vi "Run.vi"(8 "error in (no error)":errorcluster, 11 "Car Wash Station Sequencer in":refnum<class "Car Wash Station Sequencer.lvclass">) -> (0 "error out":errorcluster, 3 "Car Wash Station Sequencer out":refnum<class "Car Wash Station Sequencer.lvclass">)   [LabVIEW 2016, in "CLD Exam - Car Wash.lvlib" / "Car Wash Station Sequencer.lvclass"]
doc: "--\nCopyright © 2017 Composed SystemsI All rights reserved.\n\nAuthor: Jon McBee <jon.mcbee@composed.io>\n\nThis library is provided \"AS IS\" ,WITHOUT WARRANTIES OR\nCONDITIONS OF ANY KIND, either express or implied.\n\nComposed Systems -- composed.io\n\nStream 0.0.1.1\nJon McBee - Composed Systems\nCopyright (c) 2017, Composed Systems"
uses:
  Car Wash Station Sequencer.lvclass
  D:/Repos/Stream/software/Mediator/Classes/Mediated Actor/Mediated Actor.lvclass
  Mediator/Classes/Message Interface/Message Interface.lvclass
  Car Wash Station Sequencer.lvclass/Car Wash Station Sequencer.ctl
  Car Wash Started Event/Car Wash Started.lvclass
  Car Position Changed Event/Car Position Changed.lvclass
  Mediator/Classes/Mediated Actor/Mediated Actor.lvclass
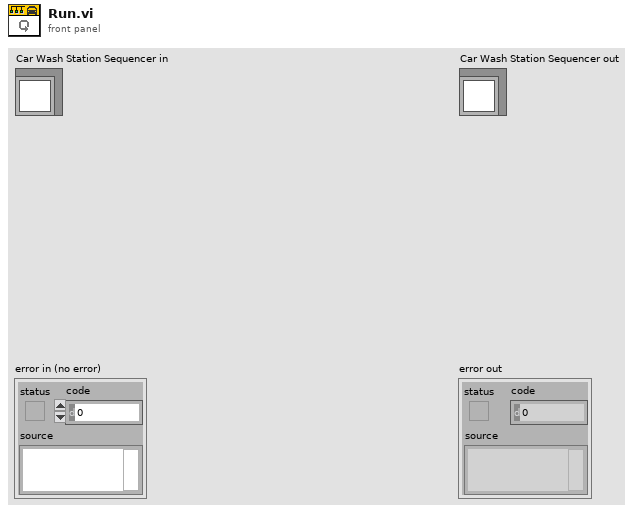
[diagram p1: front panel]
types:
  T1 = cluster{"System Exit":refnum<event-registration>, "To Self":refnum<event-registration>, "Car Wash Started":refnum<event-registration>, "Car Position Changed":refnum<event-registration>}
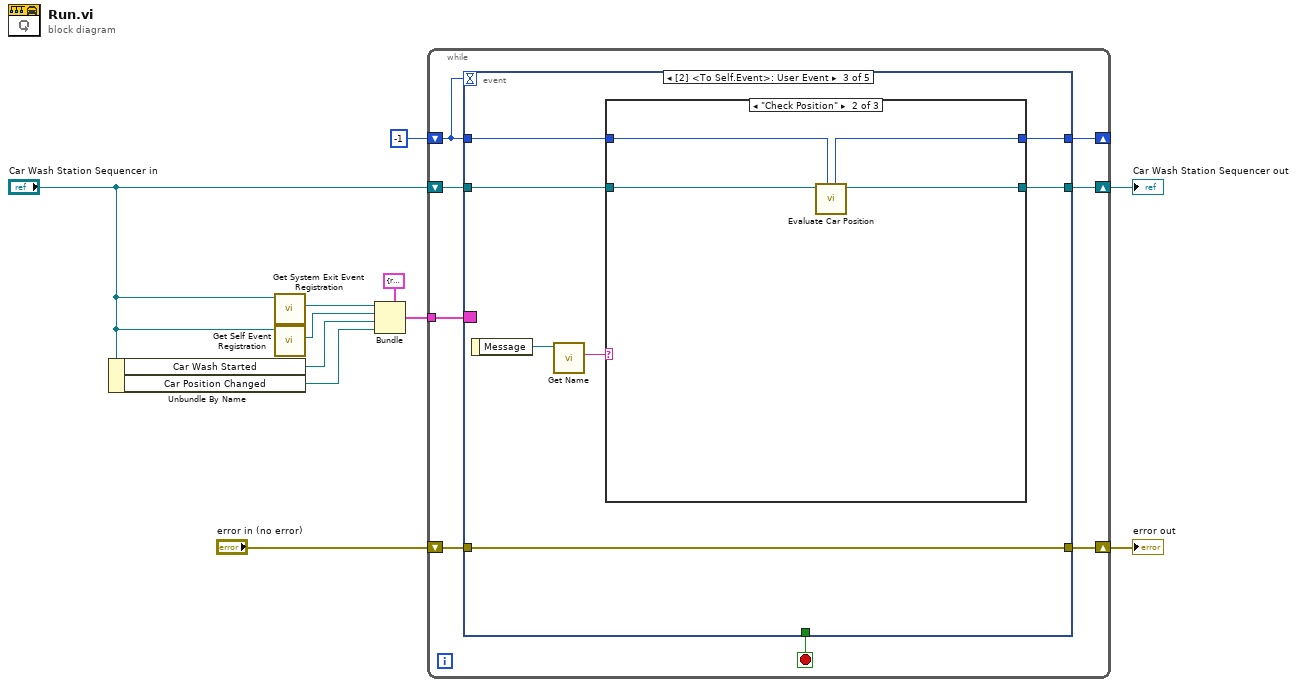
[diagram p0: block diagram]
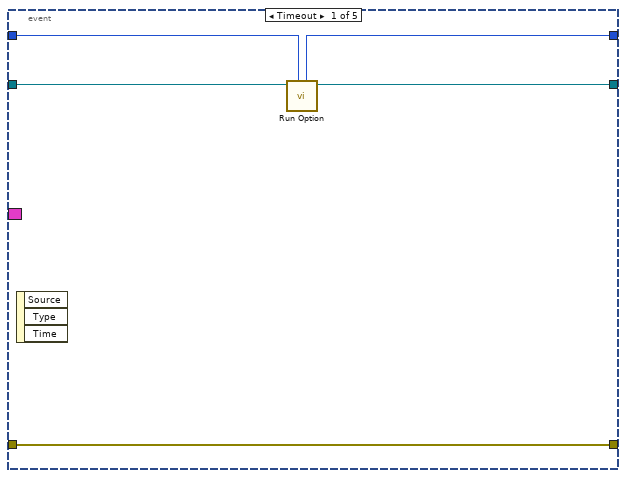
[diagram p2: hidden frame]
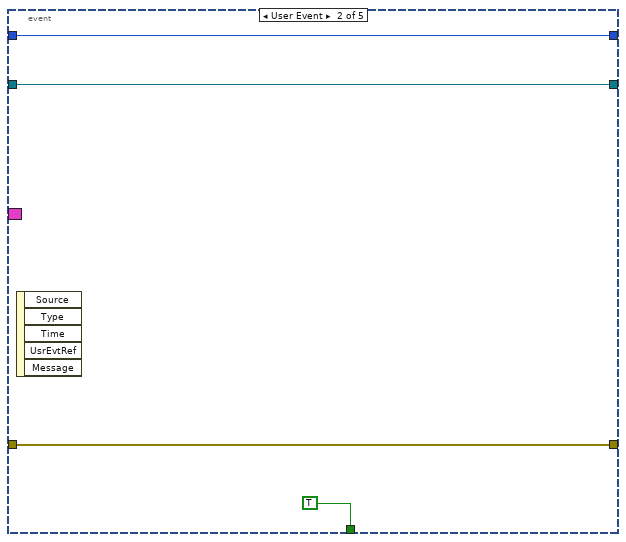
[diagram p3: hidden frame]
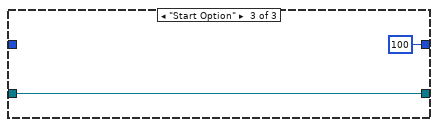
[diagram p5: hidden frame]
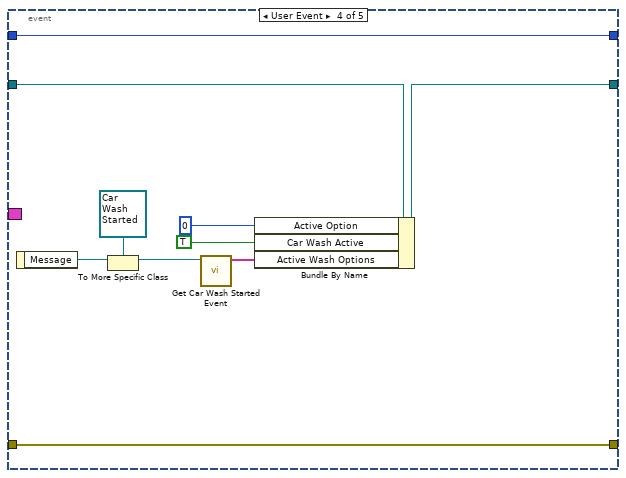
[diagram p6: hidden frame]
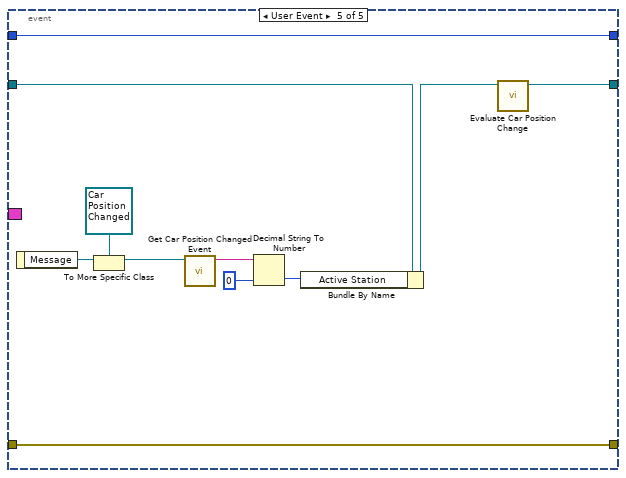
[diagram p7: hidden frame]
diagram:
  n1 = Unbundle By Name("Car Wash Station Sequencer in") -> ("Car Wash Started"=w8:refnum<event-registration>, "Car Position Changed"=w5:refnum<event-registration>)
  n2 = call "Get System Exit Event Registration.vi"("Mediated Actor in"="Car Wash Station Sequencer in") -> ("System Exit Registration"=w11:refnum<event-registration>)  [unwired: 9 in, 1 out]
  n3 = call "Get Self Event Registration.vi"("Mediated Actor in"="Car Wash Station Sequencer in") -> ("Event Registration Refnum"=w10:refnum<event-registration>)  [unwired: 9 in, 1 out]
  n4 = Bundle(cluster=T1 {"System Exit"=refnum, "To Self"=refnum, "Car Wash Started"=refnum, "Car Position Changed"=refnum} ("output cluster"), "System Exit"=w11, "To Self"=w10, "Car Wash Started"=w8, "Car Position Changed"=w5) -> (w4:T1)
  n5 = while {
    shift-right: [w18] -> w6
    shift-left: "Car Wash Station Sequencer in" -> [w19]
    tunnel: w4 -> [w17]
    shift-right: [w15] -> w2
    shift-left: "error in (no error)" -> [w16]
    shift-right: [w13] -> _
    shift-left: -1 -> [w12]
    stop <- w14 stop-if-true
    n6 = event shown="[2] <To Self.Event>: User Event" {
      selector: w17 -> [_ _ _ _ _]
      dyn-events: _ -> [_ _ _ _ _]
      timeout: w12 -> [_ _ _ _ _]
      tunnel: w19 -> [w23 w28 w33 w48 w57]
      tunnel: [w22 w28 w32 w47 w55] -> w18
      tunnel: w16 -> [w24 w27 w35 w53 w64]
      tunnel: [w24 w27 w35 w53 w64] -> w15
      tunnel: [_ TRUE _ _ _] -> w14
      tunnel: w12 -> [w21 w25 w29 w44 w54]
      tunnel: [w20 w25 w30 w44 w54] -> w13
      event Timeout {
        n7 = event-data() -> ()  [unwired: 1 in, 3 out]
        n8 = call "Run Option.vi"("Timeout"=w21, "Car Wash Station Sequencer in"=w23) -> ("Car Wash Station Sequencer out"=w22:refnum<class "Car Wash Station Sequencer.lvclass">, "Timeout out"=w20:i32)  [unwired: 8 in]
      }
      event User Event {
        n9 = event-data() -> ()  [unwired: 1 in, 5 out]
      }
      event User Event {
        n10 = event-data() -> ("Message"=w34:refnum<class "Message Interface.lvclass">)  [unwired: 1 in]
        n11 = call "Get Name.vi"("Message Interface in"=w34) -> ("Name"=w31:string)  [unwired: 8 in, 2 out]
        n12 = case shown="\"Check Position\"" w31 {
          tunnel: [w37 w40 w42] -> w32
          tunnel: w33 -> [w37 w41 w42]
          tunnel: [w36 w38 100] -> w30
          tunnel: w29 -> [w36 w39 _]
          frame Default {
          }
          frame "Check Position" {
            n13 = call "Evaluate Car Position.vi"("Timeout"=w39, "Car Wash Station Sequencer in"=w41) -> ("Car Wash Station Sequencer out"=w40:refnum<class "Car Wash Station Sequencer.lvclass">, "Timeout out"=w38:i32)  [unwired: 8 in]
          }
          frame "Start Option" {
          }
        }
      }
      event User Event {
        n14 = event-data() -> ("Message"=w52:refnum<class "Message Interface.lvclass">)  [unwired: 1 in]
        n15 = To More Specific Class(target class=refnum<class "Car Wash Started.lvclass"> refnum ("Car Wash Started.lvclass"), reference=w52) -> (specific class reference=w50:refnum<class "Car Wash Started.lvclass">)  [unwired: 1 in, 1 out]
        n16 = call "Get Car Wash Started Event.vi"("Car Wash Started in"=w50) -> ("Wash Options"=w49:string[])  [unwired: 8 in, 2 out]
        n17 = Bundle By Name(cluster=w48, "Active Option"=u8 0 ("Data.Active Option"), "Car Wash Active"=TRUE ("Data.Car Wash Active"), "Active Wash Options"=w49) -> (w47:refnum<class "Car Wash Station Sequencer.lvclass">)
      }
      event User Event {
        n18 = event-data() -> ("Message"=w63:refnum<class "Message Interface.lvclass">)  [unwired: 1 in]
        n19 = To More Specific Class(target class=refnum<class "Car Position Changed.lvclass"> refnum ("Car Position Changed.lvclass"), reference=w63) -> (specific class reference=w61:refnum<class "Car Position Changed.lvclass">)  [unwired: 1 in, 1 out]
        n20 = call "Get Car Position Changed Event.vi"("Car Position Changed in"=w61) -> ("Station"=w60:string)  [unwired: 9 in, 1 out]
        n21 = Decimal String To Number(string=w60, default (0L)=u8 0 ("default (0 I32)")) -> (number=w58:u8)  [unwired: 1 in, 1 out]
        n22 = Bundle By Name(cluster=w57, "Active Station"=w58) -> (w56:refnum<class "Car Wash Station Sequencer.lvclass">)
        n23 = call "Evaluate Car Position Change.vi"("Car Wash Station Sequencer in"=w56) -> ("Car Wash Station Sequencer out"=w55:refnum<class "Car Wash Station Sequencer.lvclass">)  [unwired: 10 in]
      }
    }
  }
  "error out" <- w2
  "Car Wash Station Sequencer out" <- w6
